vi "Defer Panel Updates.vi"(8 "error in":errorcluster, 10 "Defer Panel Updates":bool, 11 "Series UI Actor in":refnum<class "Series UI Actor.lvclass">) -> (0 "error out":errorcluster, 2 "FrontPanel Ref dup":refnum<vi>, 3 "Series UI Actor out":refnum<class "Series UI Actor.lvclass">)   [LabVIEW 2024, in "Series UI Actor.lvlib" / "Series UI Actor.lvclass"]
uses:
  Series UI Actor.lvclass
  Series UI Actor.lvclass/Series UI Actor.ctl
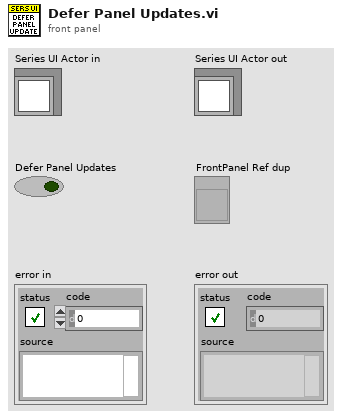
[diagram p1: front panel]
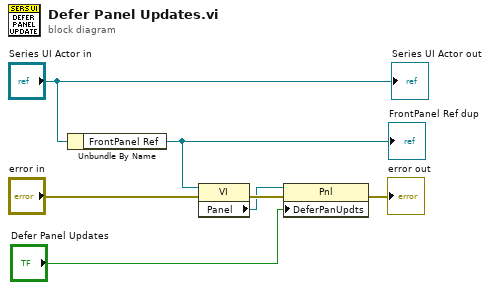
[diagram p0: block diagram]
diagram:
  n1 = Unbundle By Name("Series UI Actor in") -> ("FrontPanel Ref"=w1:refnum<vi>)
  "FrontPanel Ref dup" <- w1
  n2 = property class="VI"(reference=w1, error in="error in") -> (error out=w5:errorcluster, "Panel"=w3:refnum<vi>)  [unwired: 1 out]
  n3 = property class="Pnl"(reference=w3, error in=w5, "DeferPanUpdts"="Defer Panel Updates") -> (error out=→"error out":errorcluster)  [unwired: 1 out]
  "Series UI Actor out" <- "Series UI Actor in"
